vi "12_ВПГрафикФункции.vi"() -> ()   [LabVIEW 2016]
panel:
  out "График":dynamicdata(graph)
  in  "Вход":dbl
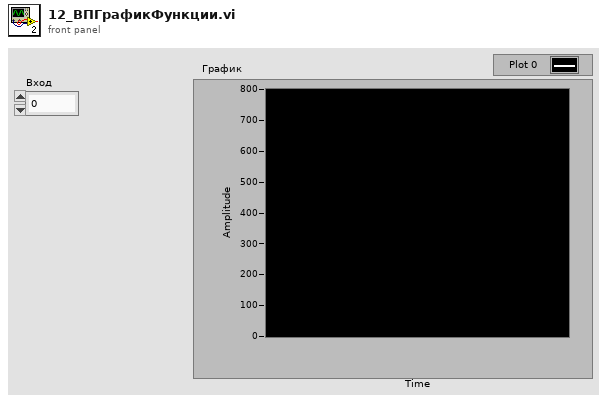
[diagram p1: front panel]
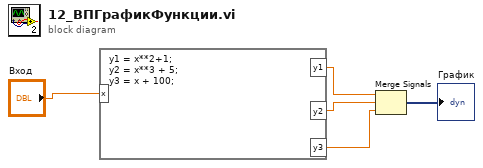
[diagram p0: block diagram]
diagram:
  n1 = formula code="y1 = x**2+1;\ny2 = x**3 + 5;\ny3 = x + 100;"("x"="Вход") -> ("y1"=w4:dbl, "y2"=w3:dbl, "y3"=w2:dbl)
  n2 = Merge Signals(w4, w3, w2) -> (→"График":dynamicdata)
